vi "sub_filter_buffer_files.vi"(8 "error in":errorcluster, 10 "Start Folder":path) -> (0 "error out":errorcluster, 2 "Output Routes and Files":T1[](array[typedef]))   [LabVIEW 2013, in "daqio minimal.lvlib"]
doc: "This VI goes through all buffer files and creates a list of files that belong to a certain API route. This way buffer files can be managed from the Buffer FGV"
uses:
  daqio minimal.lvlib
  _typedefs/daqio-Buffer-Cluster.ctl
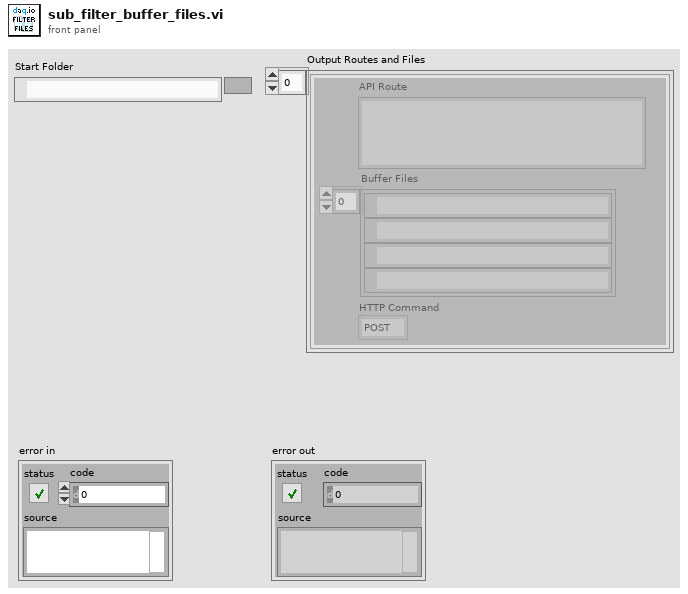
[diagram p1: front panel]
types:
  T1 = typedef "daqio minimal.lvlib/daqio-Buffer-Cluster.ctl" = cluster{"API Route":string, "Buffer Files":path[], "HTTP Command":enum16{"POST", "PUT"}}
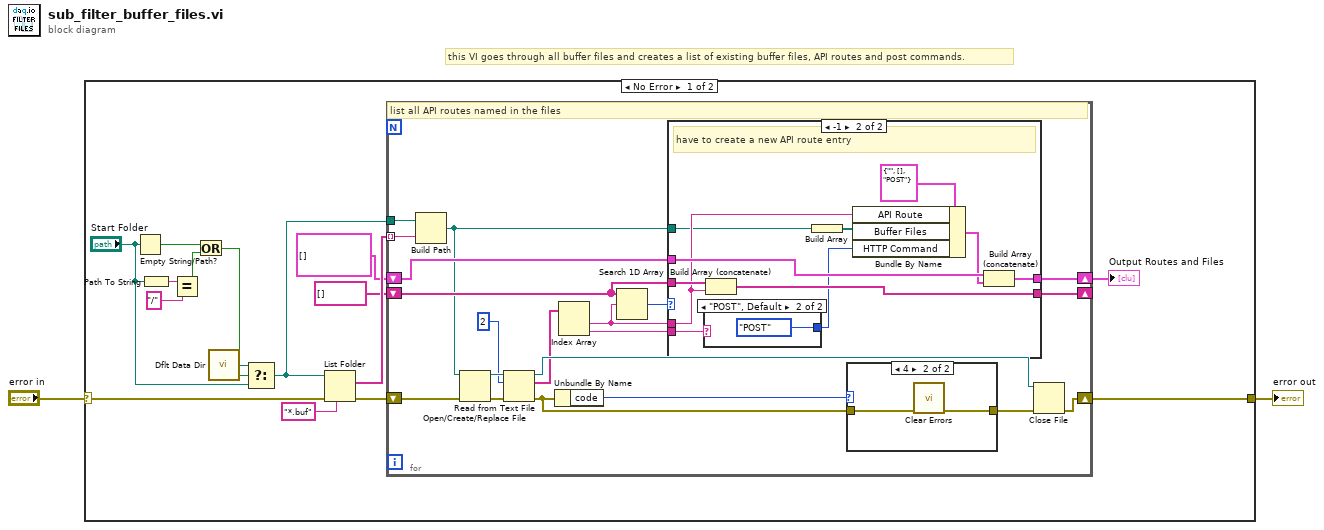
[diagram p0: block diagram]
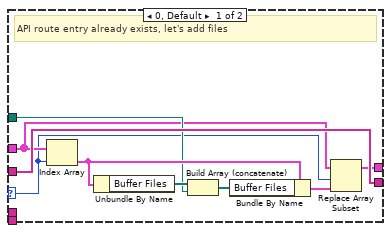
[diagram p2: hidden frame]
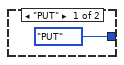
[diagram p3: hidden frame]
diagram:
  # "this VI goes through all buffer files and creates a list of existing buffer files, API routes and post commands."
  n1 = case shown="No Error" "error in" {
    selector: "error in" -> [w17 w64]
    tunnel: [w14 w64] -> w1
    frame No Error {
      n2 = Empty String/Path?(string/path="Start Folder") -> (empty?=w6:bool)
      n3 = Path To String(path="Start Folder") -> (string=w5:string)
      n4 = Equal?(x=w5, y="/") -> (x = y?=w4:bool)
      n5 = Or(x=w6, y=w4) -> (x .or. y?=w3:bool)
      n6 = call <vilib>:"Dflt Data Dir.vi"() -> ("App:Default Data Directory"=w18:path)
      n7 = Select(t=w18, s=w3, f="Start Folder") -> (s? t:f=w13:path)
      n8 = List Folder(path=w13, pattern="*.buf", error in=w17) -> (filenames=w16:string[], error out=w15:errorcluster)  [unwired: 1 in, 2 out]
      n9 = for {
        tunnel: w16 -> [w29] mode=indexing
        shift-right: [w30] -> w14
        shift-left: w15 -> [w34]
        tunnel: w13 -> [w28]
        shift-right: [w24] -> _
        shift-left: string[] [] -> [w25]
        shift-right: [w20] -> w10
        shift-left: T1[] [] -> [w22]
        # "list all API routes named in the files"
        n10 = Build Path(base path=w28, name or relative path=w29) -> (appended path=w21:path)
        n11 = Open/Create/Replace File(file path (use dialog)=w21, error in=w34) -> (refnum out=w38:refnum<file>, error out=w35:errorcluster)  [unwired: 4 in, 1 out]
        n12 = Read from Text File(file (use dialog)=w38, count=2, error in=w35) -> (refnum out=w31:refnum<file>, text=w27:string[], error out=w36:errorcluster)  [unwired: 1 in, 1 out]
        n13 = Unbundle By Name(w36) -> ("code"=w37:i32)
        n14 = Index Array(array=w27) -> (element #1=w23:string, element #2=w19:string)  [unwired: 2 in]
        n15 = Search 1D Array(1D array=w25, element=w23) -> (index of element=w26:i32)  [unwired: 1 in]
        n16 = case shown="-1" w26 {
          selector: w26 -> [w41 _]
          tunnel: w25 -> [w47 w58]
          tunnel: [w47 w57] -> w24
          tunnel: w23 -> [_ w55]
          tunnel: w22 -> [w42 w56]
          tunnel: w21 -> [w44 w54]
          tunnel: [w39 w52] -> w20
          tunnel: w19 -> [_ w49]
          frame 0, Default {
            # "API route entry already exists, let's add files"
            n17 = Index Array(array=w42, index=w41) -> (element=w46:T1)
            n18 = Unbundle By Name(w46) -> ("Buffer Files"=w45:path[])
            n19 = Build Array (concatenate)(w45, w44) -> (w43:path[])
            n20 = Bundle By Name(cluster=w46, "Buffer Files"=w43) -> (w40:T1)
            n21 = Replace Array Subset(array=w42, new element=w40, index=w41) -> (w39:T1[])
          }
          frame -1 {
            # "have to create a new API route entry"
            n22 = case shown="\"POST\", Default" w49 {
              tunnel: [enum16{"POST", "PUT"}."PUT" ("HTTP Command") enum16{"POST", "PUT"}."POST" ("HTTP Command")] -> w48
              frame "PUT" {
              }
              frame "POST", Default {
              }
            }
            n23 = Build Array (concatenate)(w58, w55) -> (w57:string[])
            n24 = Build Array(w54) -> (w53:path[])
            n25 = Bundle By Name(cluster=T1 {"API Route"="", "Buffer Files"=[], "HTTP Command"=enum."POST"} ("Buffer Cluster"), "API Route"=w55, "Buffer Files"=w53, "HTTP Command"=w48) -> (w51:T1)
            n26 = Build Array (concatenate)(w56, w51) -> (w52:T1[])
          }
        }
        n27 = case shown="4" w37 {
          tunnel: w36 -> [w61 w63]
          tunnel: [w61 w62] -> w32
          frame 0, Default {
          }
          frame 4 {
            n28 = call <vilib>:"Clear Errors.vi"("error in (no error)"=w63) -> ("error out"=w62:errorcluster)  [unwired: 6 in]
          }
        }
        n29 = Close File(refnum=w31, error in=w32) -> (error out=w30:errorcluster)  [unwired: 1 out]
      }
      "Output Routes and Files" <- w10
    }
    frame Error {
    }
  }
  "error out" <- w1
